vi "Set_Names_ID_Samples.vi"(8 "error in (no error)":errorcluster, 11 "DB in":refnum<class "DB.lvclass">) -> (0 "error out":errorcluster, 3 "DB out":refnum<class "DB.lvclass">)   [LabVIEW 2019, in "DB.lvclass"]
uses:
  DB.lvclass
  DB.lvclass/DB.ctl
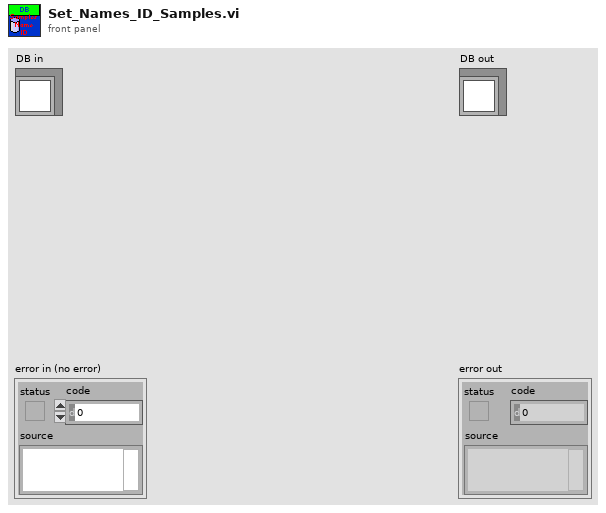
[diagram p1: front panel]
types:
  T1 = typedef "DB.lvclass/Def_fix_sql_param.ctl" = cluster{"Fix Project":bool, "Fix Sample":bool, "Fix Exp Date":bool, "Fix User":bool}
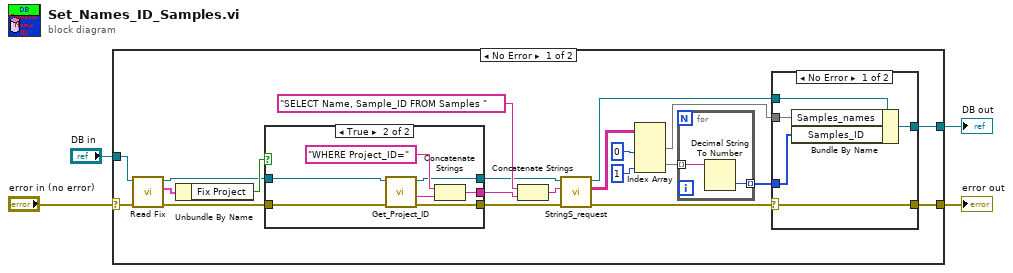
[diagram p0: block diagram]
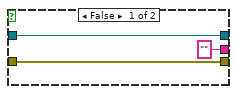
[diagram p2: hidden frame]
diagram:
  n1 = case shown="No Error" "error in (no error)" {
    selector: "error in (no error)" -> [w14 w46]
    tunnel: [w16 w46] -> w3
    tunnel: [w17 w45] -> w1
    tunnel: "DB in" -> [w15 w45]
    frame No Error {
      n2 = call "Read Fix.vi"("error in (no error)"=w14, "DB in"=w15) -> ("error out"=w7:errorcluster, "Fix"=w13:T1, "DB out"=w9:refnum<class "DB.lvclass">)  [unwired: 7 in]
      n3 = Unbundle By Name(w13) -> ("Fix Project"=w12:bool)
      n4 = case shown="True" w12 {
        tunnel: ["" w34] -> w11
        tunnel: w9 -> [w28 w33]
        tunnel: [w28 w31] -> w8
        tunnel: w7 -> [w27 w30]
        tunnel: [w27 w29] -> w6
        frame False {
        }
        frame True {
          n5 = call "Get_Project_ID.vi"("error in (no error)"=w30, "DB in"=w33) -> ("error out"=w29:errorcluster, "Project_ID"=w32:string, "DB out"=w31:refnum<class "DB.lvclass">)  [unwired: 6 in, 1 out]
          n6 = Concatenate Strings("WHERE Project_ID=", w32) -> (w34:string)
        }
      }
      n7 = Concatenate Strings("SELECT Name, Sample_ID FROM Samples " ("SQL"), w11) -> (w5:string)
      n8 = call-dynamic "StringS_request.vi"("error in (no error)"=w6, "SQL request"=w5, "DB in"=w8) -> ("error out"=w23:errorcluster, "Result Set"=w21:string[][], "DB out"=w25:refnum<class "DB.lvclass">)  [unwired: 5 in, 1 out]
      n9 = Index Array(array=w21, index (col) #1=0 ("disabled index (col)"), index (col) #2=1 ("index (col)")) -> (element #1=w24:string[], element #2=w20:string[])  [unwired: 2 in]
      n10 = for {
        tunnel: w20 -> [w44] mode=indexing
        tunnel: [w43] -> w22 mode=indexing
        n11 = Decimal String To Number(string=w44) -> (number=w43:i32)  [unwired: 2 in, 1 out]
      }
      n12 = case shown="No Error" w23 {
        selector: w23 -> [w36 w41]
        tunnel: w25 -> [w40 w42]
        tunnel: [w39 w42] -> w17
        tunnel: w22 -> [w38 _]
        tunnel: w24 -> [w37 _]
        tunnel: [w36 w41] -> w16
        frame No Error {
          n13 = Bundle By Name(cluster=w40, "Samples_names"=w37, "Samples_ID"=w38) -> (w39:refnum<class "DB.lvclass">)
        }
        frame Error {
        }
      }
    }
    frame Error {
    }
  }
  "error out" <- w3
  "DB out" <- w1
